vi "Get bcd usb.vi"(8 "error in":errorcluster caption="エラー入力", 10 "PID":i32=33 format="%04x", 11 "VID":i32=9472 format="%04x") -> (0 "error out":errorcluster caption="エラー出力", 3 "BcdUsb":i16 format="%04x")   [LabVIEW 2020]
uses:
  C:/Users/Mikio Fukushima/Desktop/work/LibUsbDotNet/fs-dotnet/fs-dotnet/LabVIEW/LibUsbDotNet.dll
  LibUsbDotNet.dll
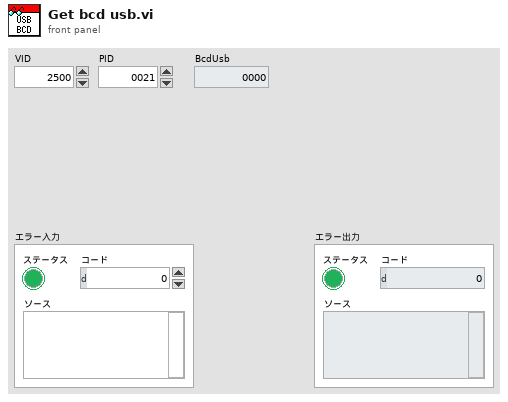
[diagram p1: front panel]
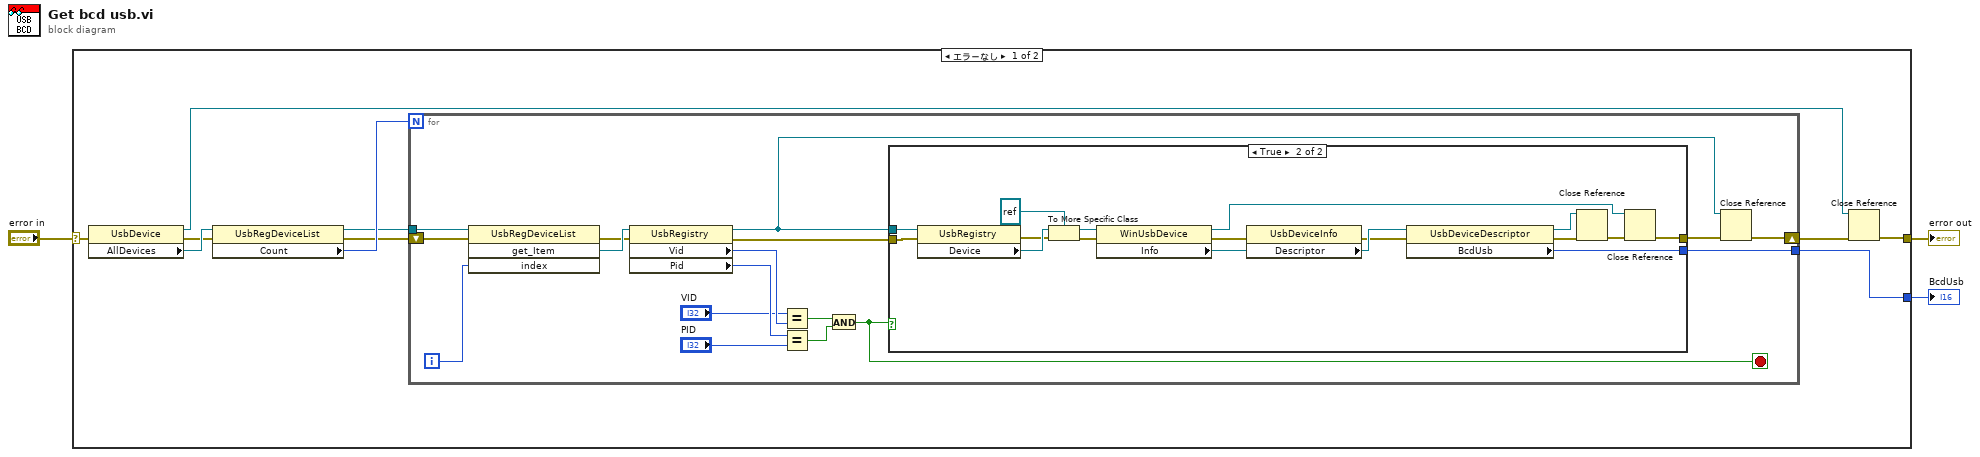
[diagram p0: block diagram]
diagram:
  n1 = case shown="エラーなし" "error in" {
    selector: "error in" -> [w5 w49]
    tunnel: [w9 _] -> w3
    tunnel: [w4 w49] -> w1
    frame No Error {
      n2 = property on="プロパティノード" class="UsbDevice"(error in=w5) -> (reference out=w6:refnum<k24>, error out=w10:errorcluster, "AllDevices"=w13:refnum<k24>)  [unwired: 1 in]
      n3 = property on="プロパティノード" class="UsbRegDeviceList"(reference=w13, error in=w10) -> (reference out=w11:refnum<k24>, error out=w8:errorcluster, "Count"=w12:i32)
      n4 = for {
        N: w12 -> [_]
        tunnel: w11 -> [w30]
        tunnel: [w18] -> w9
        shift-right: [w14] -> w7
        shift-left: w8 -> [w17]
        i -> [w29]
        stop <- w21 stop-if-true
        n5 = invoke on="インボークノード" class="UsbRegDeviceList" method="get_Item"(reference=w30, error in=w17, "index"=w29) -> (error out=w20:errorcluster, "get_Item"=w28:refnum<k24>)  [unwired: 1 in, 2 out]
        n6 = property on="プロパティノード" class="UsbRegistry"(reference=w28, error in=w20) -> (reference out=w16:refnum<k24>, error out=w19:errorcluster, "Vid"=w26:i32, "Pid"=w27:i32)
        n7 = Equal?(x="VID", y=w26) -> (x = y?=w23:bool)
        n8 = Equal?(x=w27, y="PID") -> (x = y?=w22:bool)
        n9 = And(x=w23, y=w22) -> (x .and. y?=w21:bool)
        n10 = case shown="TRUE" w21 {
          tunnel: w16 -> [_ w48]
          tunnel: w19 -> [w31 w38]
          tunnel: [_ w37] -> w18
          tunnel: [w31 w32] -> w15
          frame False {
          }
          frame True {
            n11 = property on="プロパティノード" class="UsbRegistry"(reference=w48, error in=w38) -> (error out=w39:errorcluster, "Device"=w47:refnum<k24>)  [unwired: 1 out]
            n12 = To More Specific Class(target class=refnum<k24> refnum ("リファレンス出力"), reference=w47, error in=w39) -> (specific class reference=w45:refnum<k24>, error out=w40:errorcluster)
            n13 = property on="プロパティノード" class="WinUsbDevice"(reference=w45, error in=w40) -> (reference out=w34:refnum<k24>, error out=w41:errorcluster, "Info"=w44:refnum<k24>)
            n14 = property on="プロパティノード" class="UsbDeviceInfo"(reference=w44, error in=w41) -> (error out=w42:errorcluster, "Descriptor"=w43:refnum<k24>)  [unwired: 1 out]
            n15 = property on="プロパティノード" class="UsbDeviceDescriptor"(reference=w43, error in=w42) -> (reference out=w35:refnum<k24>, error out=w36:errorcluster, "BcdUsb"=w37:i16)
            n16 = Close Reference(reference=w35, error in (no error)=w36) -> (error out=w33:errorcluster)
            n17 = Close Reference(reference=w34, error in (no error)=w33) -> (error out=w32:errorcluster)
          }
        }
        n18 = Close Reference(reference=w16, error in (no error)=w15) -> (error out=w14:errorcluster)
      }
      n19 = Close Reference(reference=w6, error in (no error)=w7) -> (error out=w4:errorcluster)
    }
    frame Error {
    }
  }
  "BcdUsb" <- w3
  "error out" <- w1
